vi "sampleCalculator.vi"() -> ()   [LabVIEW 2018]
panel:
  in  "stop":bool
  out "Display":string
  in  "2":bool
  in  "1":bool
  in  "minus":bool
  in  "plus":bool
  in  "equal":bool
  in  "C":bool
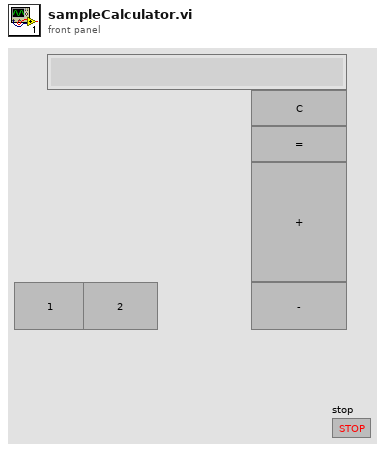
[diagram p1: front panel]
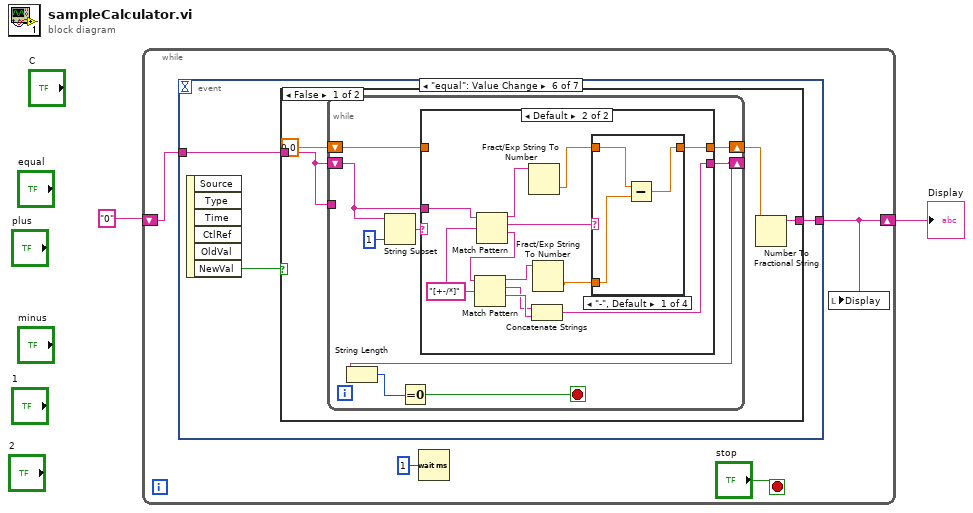
[diagram p0: block diagram]
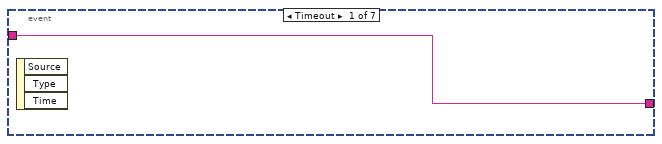
[diagram p2: hidden frame]
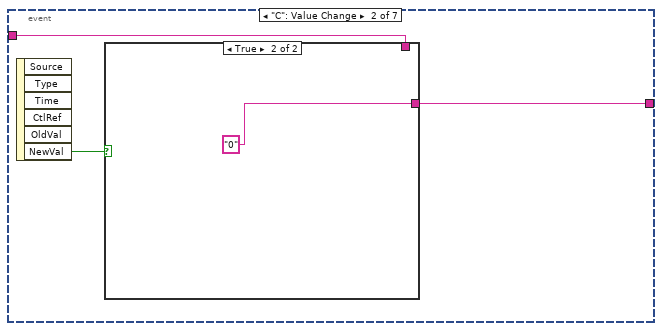
[diagram p3: hidden frame]
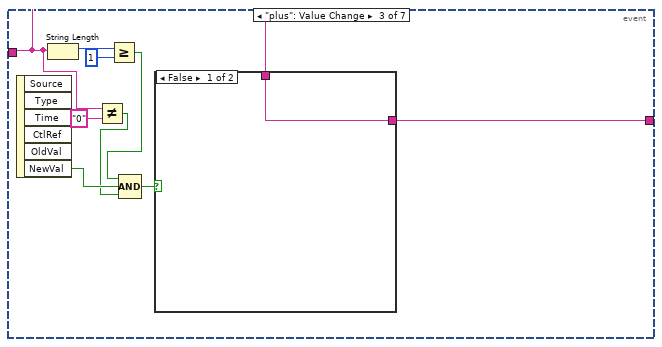
[diagram p5: hidden frame]
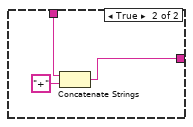
[diagram p6: hidden frame]
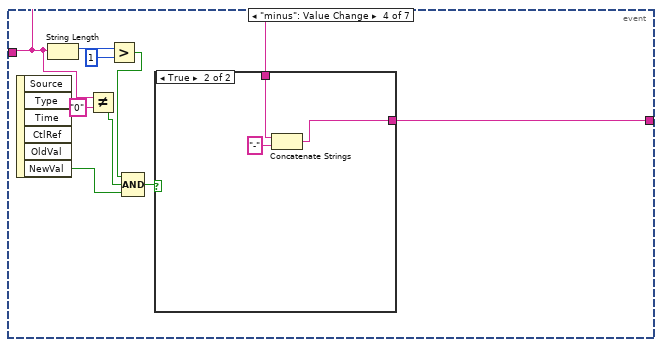
[diagram p7: hidden frame]
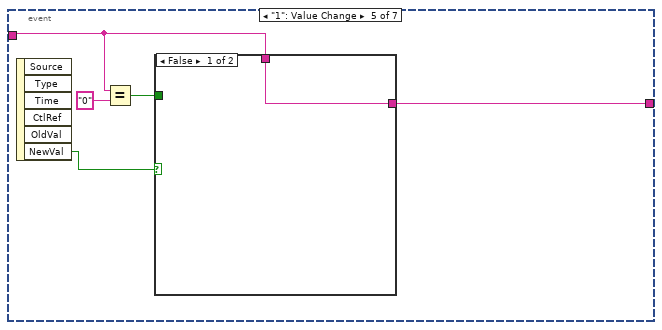
[diagram p9: hidden frame]
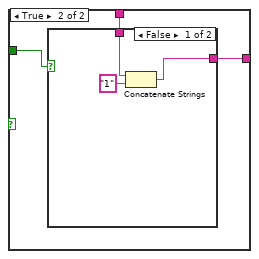
[diagram p10: hidden frame]
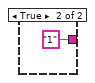
[diagram p11: hidden frame]
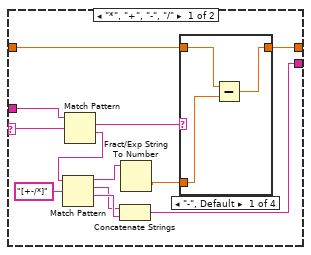
[diagram p12: hidden frame]
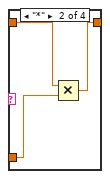
[diagram p13: hidden frame]
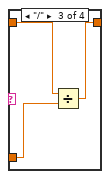
[diagram p14: hidden frame]
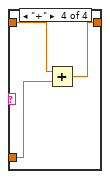
[diagram p15: hidden frame]
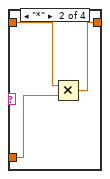
[diagram p16: hidden frame]
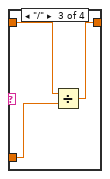
[diagram p17: hidden frame]
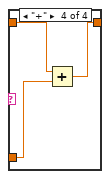
[diagram p18: hidden frame]
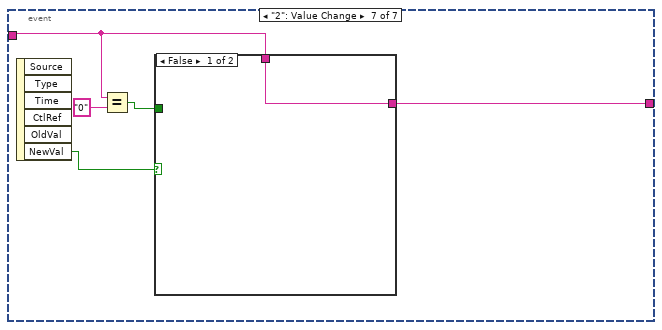
[diagram p20: hidden frame]
diagram:
  n1 = while {
    shift-right: [w3] -> w1
    shift-left: "0" ("Display") -> [w5]
    stop <- "stop" stop-if-true
    n2 = event shown="[5] \"equal\": Value Change" {
      selector: _ -> [_ _ _ _ _ _ _]
      dyn-events: _ -> [_ _ _ _ _ _ _]
      timeout: _ -> [_ _ _ _ _ _ _]
      tunnel: w5 -> [w7 w8 w18 w28 w41 w52 w118]
      tunnel: [w7 w9 w19 w32 w43 w54 w120] -> w3
      event Timeout {
        n3 = event-data() -> ()  [unwired: 1 in, 3 out]
      }
      event "C": Value Change {
        n4 = event-data() -> ("NewVal"=w10:bool)  [unwired: 1 in, 5 out]
        n5 = case shown="True" w10 {
          tunnel: [w11 "0" ("Display")] -> w9
          tunnel: w8 -> [w11 _]
          frame False {
          }
          frame True {
          }
        }
      }
      event "plus": Value Change {
        n6 = event-data() -> ("NewVal"=w14:bool)  [unwired: 1 in, 5 out]
        n7 = String Length(string=w18) -> (length=w21:i32)
        n8 = Not Equal?(x=w18, y="0") -> (x != y?=w13:bool)
        n9 = Greater Or Equal?(x=w21, y=1) -> (x >= y?=w15:bool)
        n10 = Compound Arithmetic op=AND(w15, w14, w13) -> (w16:bool)
        n11 = case shown="False" w16 {
          tunnel: w18 -> [w22 w25]
          tunnel: [w22 w23] -> w19
          frame False {
          }
          frame True {
            n12 = Concatenate Strings(w25, "+" ("string")) -> (w23:string)
          }
        }
      }
      event "minus": Value Change {
        n13 = event-data() -> ("NewVal"=w29:bool)  [unwired: 1 in, 5 out]
        n14 = String Length(string=w28) -> (length=w34:i32)
        n15 = Not Equal?(x=w28, y="0") -> (x != y?=w26:bool)
        n16 = Greater?(x=w34, y=1) -> (0:w30:bool)
        n17 = Compound Arithmetic op=AND(w30, w26, w29) -> (w31:bool)
        n18 = case shown="True" w31 {
          tunnel: w28 -> [w35 w38]
          tunnel: [w35 w36] -> w32
          frame False {
          }
          frame True {
            n19 = Concatenate Strings(w38, "-" ("string")) -> (w36:string)
          }
        }
      }
      event "1": Value Change {
        n20 = event-data() -> ("NewVal"=w42:bool)  [unwired: 1 in, 5 out]
        n21 = Equal?(x=w41, y="0") -> (x = y?=w39:bool)
        n22 = case shown="False" w42 {
          tunnel: w41 -> [w44 w47]
          tunnel: [w44 w46] -> w43
          tunnel: w39 -> [_ w45]
          frame False {
          }
          frame True {
            n23 = case shown="False" w45 {
              tunnel: w47 -> [w50 _]
              tunnel: [w48 "1"] -> w46
              frame False {
                n24 = Concatenate Strings(w50, "1" ("string")) -> (w48:string)
              }
              frame True {
              }
            }
          }
        }
      }
      event "equal": Value Change {
        n25 = event-data() -> ("NewVal"=w53:bool)  [unwired: 1 in, 5 out]
        n26 = case shown="False" w53 {
          tunnel: [w57 w115] -> w54
          tunnel: w52 -> [w55 w115]
          frame False {
            n27 = while {
              tunnel: w55 -> [_]
              shift-right: [w62] -> w56
              shift-left: 0.0 -> [w61]
              shift-right: [w59] -> _
              shift-left: w55 -> [w60]
              stop <- w65 stop-if-true
              n28 = String Subset(string=w60, length (rest)=1 ("length (rest)")) -> (substring=w63:string)  [unwired: 1 in]
              n29 = case shown="Default" w63 {
                selector: w63 -> [w78 _]
                tunnel: w60 -> [w77 w102]
                tunnel: [w71 w97] -> w59
                tunnel: [w68 w94] -> w62
                tunnel: w61 -> [w67 _]
                frame "*", "+", "-", "/" {
                  n30 = Match Pattern(string=w77, regular expression=w78) -> (match substring=w70:string, after substring=w76:string)  [unwired: 1 in, 2 out]
                  n31 = Match Pattern(string=w76, regular expression="[+-/*]") -> (before substring=w74:string, match substring=w72:string, after substring=w73:string)  [unwired: 1 in, 1 out]
                  n32 = Concatenate Strings(w72, w73) -> (w71:string)
                  n33 = Fract/Exp String To Number(string=w74) -> (number=w69:dbl)  [unwired: 3 in, 1 out]
                  n34 = case shown="\"-\", Default" w70 {
                    tunnel: w69 -> [w81 w84 w87 w90]
                    tunnel: [w79 w82 w86 w88] -> w68
                    tunnel: w67 -> [w80 w83 w85 w89]
                    frame "-", Default {
                      n35 = Subtract(x=w80, y=w81) -> (x-y=w79:dbl)
                    }
                    frame "*" {
                      n36 = Multiply(x=w83, y=w84) -> (x*y=w82:dbl)
                    }
                    frame "/" {
                      n37 = Divide(x=w85, y=w87) -> (x/y=w86:dbl)
                    }
                    frame "+" {
                      n38 = Add(x=w89, y=w90) -> (x+y=w88:dbl)
                    }
                  }
                }
                frame Default {
                  w91 = "[+-/*]" ("regular expression")
                  n39 = Match Pattern(string=w102, regular expression=w91) -> (before substring=w93:string, match substring=w96:string, after substring=w101:string)  [unwired: 1 in, 1 out]
                  n40 = Match Pattern(string=w101, regular expression=w91) -> (before substring=w100:string, match substring=w98:string, after substring=w99:string)  [unwired: 1 in, 1 out]
                  n41 = Fract/Exp String To Number(string=w93) -> (number=w92:dbl)  [unwired: 3 in, 1 out]
                  n42 = Concatenate Strings(w98, w99) -> (w97:string)
                  n43 = Fract/Exp String To Number(string=w100) -> (number=w95:dbl)  [unwired: 3 in, 1 out]
                  n44 = case shown="\"-\", Default" w96 {
                    tunnel: w95 -> [w105 w108 w111 w114]
                    tunnel: [w103 w106 w110 w112] -> w94
                    tunnel: w92 -> [w104 w107 w109 w113]
                    frame "-", Default {
                      n45 = Subtract(x=w104, y=w105) -> (x-y=w103:dbl)
                    }
                    frame "*" {
                      n46 = Multiply(x=w107, y=w108) -> (x*y=w106:dbl)
                    }
                    frame "/" {
                      n47 = Divide(x=w109, y=w111) -> (x/y=w110:dbl)
                    }
                    frame "+" {
                      n48 = Add(x=w113, y=w114) -> (x+y=w112:dbl)
                    }
                  }
                }
              }
              n49 = String Length(string=w59) -> (length=w66:i32)
              n50 = Equal To 0?(x=w66) -> (x = 0?=w65:bool)
            }
            n51 = Number To Fractional String(number=w56) -> (F-format string=w57:string)  [unwired: 3 in]
          }
          frame True {
          }
        }
      }
      event "2": Value Change {
        n52 = event-data() -> ("NewVal"=w119:bool)  [unwired: 1 in, 5 out]
        n53 = Equal?(x=w118, y="0") -> (x = y?=w116:bool)
        n54 = case shown="False" w119 {
          tunnel: w118 -> [w121 w124]
          tunnel: [w121 w123] -> w120
          tunnel: w116 -> [_ w122]
          frame False {
          }
          frame True {
            n55 = case shown="True" w122 {
              tunnel: w124 -> [w127 _]
              tunnel: [w125 "2"] -> w123
              frame False {
                n56 = Concatenate Strings(w127, "2" ("string")) -> (w125:string)
              }
              frame True {
              }
            }
          }
        }
      }
    }
    n57 = Wait (ms)(milliseconds to wait=u32 1) -> ()  [unwired: 1 out]
    n58 = local write "Display"(w3) -> ()
  }
  "Display" <- w1
